vi "Event Last Ack.vi"(10 "Event Actor":refnum<class "Event Actor.lvclass">, 11 "Event Last Ack in":refnum<class "Event Last Ack.lvclass">) -> (3 "Event Last Ack out":refnum<class "Event Last Ack.lvclass">)   [LabVIEW 2021, in "jettl.lvlib" / "Event Last Ack.lvlib" / "Event Last Ack.lvclass"]
uses:
  Event Last Ack.lvclass
  Actor/Event Actor/Event Actor.lvclass
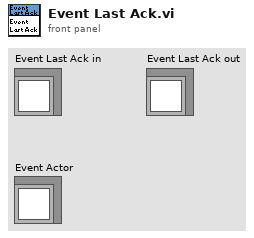
[diagram p1: front panel]
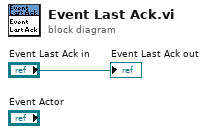
[diagram p0: block diagram]
diagram:
  "Event Last Ack out" <- "Event Last Ack in"
